vi "Config.vi"(8 "error in (no error)":errorcluster, 11 "System Actor in":refnum<class "System Actor.lvclass">) -> (0 "error out":errorcluster, 3 "System Actor out":refnum<class "System Actor.lvclass">)   [LabVIEW 2014, in "Robot Actor Framework.lvlib" / "System Actor.lvlib" / "System Actor.lvclass"]
uses:
  System Actor.lvclass
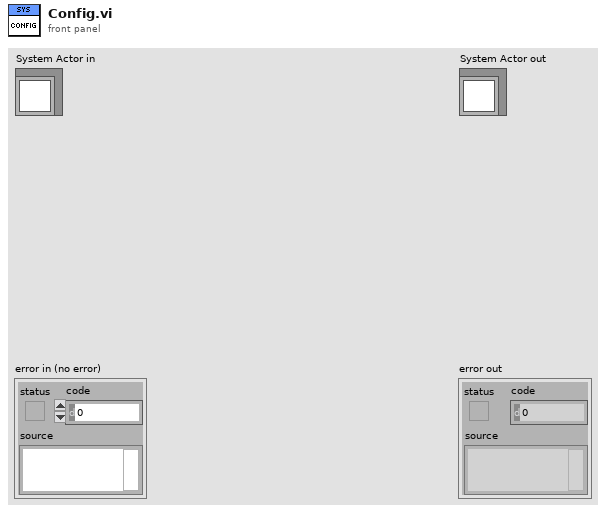
[diagram p1: front panel]
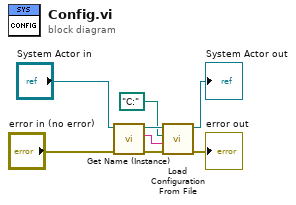
[diagram p0: block diagram]
diagram:
  n1 = call-dynamic "Get Name (Instance).vi"("error in (no error)"="error in (no error)", "System Actor in"="System Actor in") -> ("error out"=w4:errorcluster, "System Name - Instance"=w1:string, "System Actor out"=w8:refnum<class "System Actor.lvclass">)  [unwired: 7 in]
  n2 = call-dynamic "Load Configuration From File.vi"("error in (no error)"=w4, "Name (Instance)"=w1, "Configuration Path"=path "C:", "System Actor in"=w8) -> ("error out"=→"error out":errorcluster, "System Actor out"=→"System Actor out":refnum<class "System Actor.lvclass">)  [unwired: 5 in, 1 out]
